vi "Main_for_Motor_Sim.vi"() -> ()   [LabVIEW 2017]
panel:
  in  "Cluster":cluster{"b":dbl, "a2":dbl, "a1":dbl, "a0":dbl}={"b"=0.3334, "a2"=0.0052, "a1"=0.1894, "a0"=0.0}
  out "Waveform Chart":cluster{"Signal Output":dbl, "Position":dbl}(graph)
  in  "Delay (ms)":i32=10
  in  "dt":dbl=0.01
  in  "Frequency":dbl=1.0
  in  "Amplitude":dbl=1.0
  in  "Signal type":u16(ring) items=["Sinusoidal", "Triangle", "Square"]
  in  "stop":bool
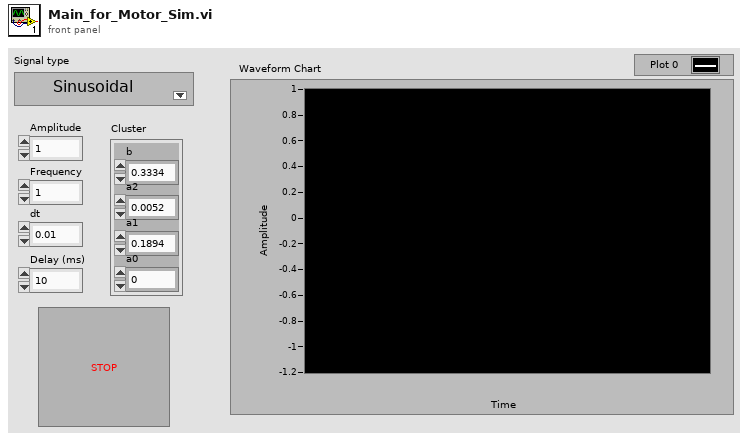
[diagram p1: front panel]
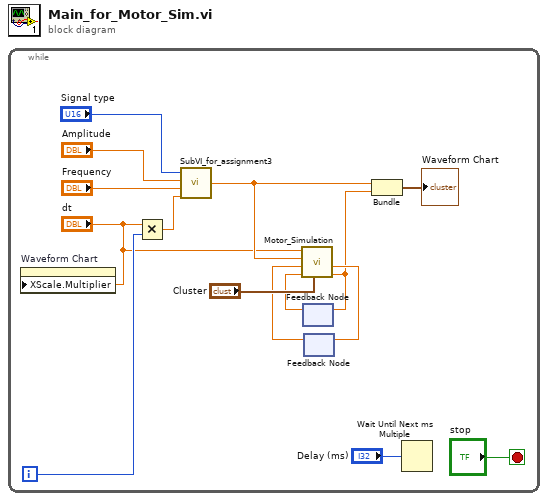
[diagram p0: block diagram]
diagram:
  n1 = while {
    i -> [w14]
    stop <- "stop" stop-if-true
    n2 = property on="Waveform Chart" class="WFChart (strict)"("XScale.Multiplier"="dt") -> ()  [unwired: 2 in, 2 out]
    n3 = Multiply(x="dt", y=w14) -> (x*y=w9:dbl)
    n4 = call "SubVI_for_assignment3.vi"("Time interval"=w9, "Frequency"="Frequency", "Amplitude"="Amplitude", "Signal type"="Signal type") -> ("Signal Output"=w3:dbl)
    n5 = feedback #1() -> (w6:dbl)  [unwired: 1 in]
    n6 = feedback #2() -> (w4:dbl)  [unwired: 1 in]
    n7 = call "Motor_Simulation.vi"("Cluster"="Cluster", "Position"=w6, "Velocity"=w4, "Input (Vm)"=w3, "dt"="dt") -> ("Position"=w1:dbl, "Velocity"=w5:dbl)  [unwired: 5 in]
    n8 = feedback-in #1(w1) -> ()
    n9 = feedback-in #2(w5) -> ()
    n10 = Bundle("Signal Output"=w3, "Position"=w1) -> (→"Waveform Chart":cluster{"Signal Output":dbl, "Position":dbl})  [unwired: 1 in]
    n11 = Wait Until Next ms Multiple(millisecond multiple="Delay (ms)") -> ()  [unwired: 1 out]
  }
